vi "iRFMeasureAuto.vi"() -> ()   [LabVIEW 2019]
uses:
  SubVI/LabJack/LJ Pin Setting.ctl
  SubVI/LabJack/LJ PWM Setting.ctl
  <instrlib>/niScope/Controls/niScope vertical coupling.ctl
  <instrlib>/niScope/Controls/niScope trigger source.ctl
  <vilib>/Analysis/baseanly.llb/Mean (DBL).vi
  <instrlib>/niScope/Configure/Trigger/niScope Configure Trigger Edge.vi
  <instrlib>/niScope/Acquire/Fetch/niScope Fetch.vi
  <instrlib>/niScope/Acquire/Fetch/niScope Multi Fetch.vi
  <vilib>/Analysis/NI_AALBase.lvlib
panel:
  in  "Prefix":string
  out "Current State":string
  out "Exit Try":bool
  in  "Suffix":string
  out "355nm Laser":bool
  out "laser EM lamp V":dbl format="%0.6f"
  in  "Aquire":bool
  in  "Current V":dbl min=0.0 max=4.7 step=0.1
  out "error out":errorcluster
  in  "Live":bool=TRUE
  out "Waveform Graph":dbl[](graph)
  in  "Channel":enum16{"Ch1", "Ch2", "Ch3"}(ring)
  in  "OK":bool
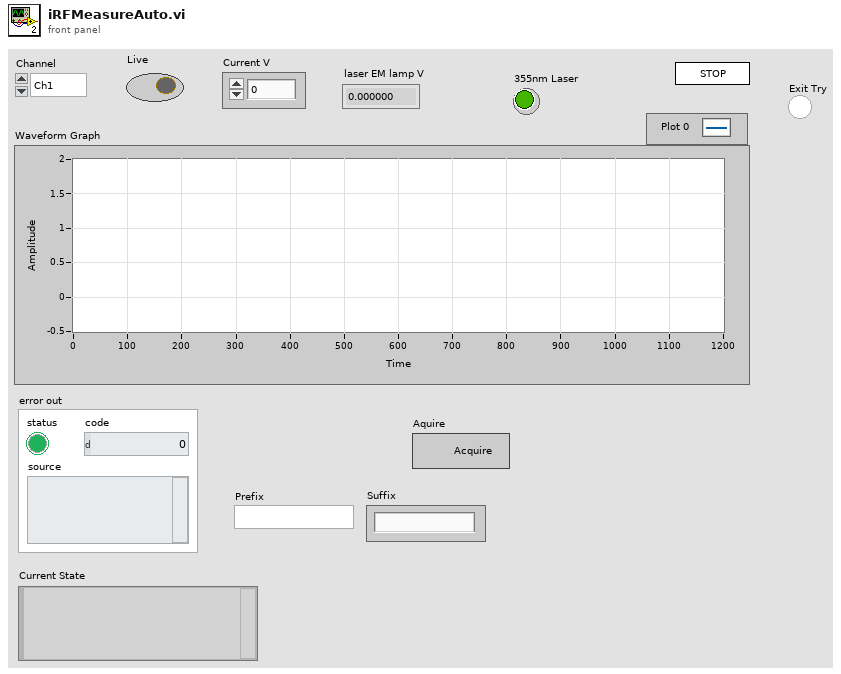
[diagram p1: front panel]
types:
  T1 = enum32{"Invalid", "Standard", "Closed", "Hidden", "Minimized", "Maximized"}
  T2 = enum32{"invalid app kind", "Development System", "Run Time System", "Student Edition", "Embedded LabVIEW", "Evaluation", "Custom"}
  T3 = typedef "niScope trigger source.ctl" = string
  T4 = enum16{"open", "open or create", "create or replace", "create", "open (read-only)"}
  T5 = typedef "LJ Pin Setting.ctl" = cluster{"Ch1 Bias":string, "Ch2 Bias":string, "Ch3 Bias":string, "355 PWM":string, "AimingBeam PWM":string, "Laser Ready":string, "Interlock":string, "Laser Start/Stop":string, "Red LED":string, "Green LED":string, "Foot Pedal":string}
  T6 = typedef "LJ PWM Setting.ctl" = cluster{"DIO_EF_CLOCK1_DIVISOR":i16, "DIO_EF_CLOCK1_ROLL_VALUE":i32, "DIO#_EF_INDEX":i16, "DIO#_EF_OPTIONS":i16, "DIO#_EF_CONFIG_A":i32}
  T7 = cluster{"Core":cluster{"Current VI Reference":refnum<vi>, "Close Panel on Exit?":bool}, "355 Status":bool, "Your string data":string, "Channel":enum16{"Ch1", "Ch2", "Ch3"}, "Digitizer":refnum<k15>, "Dig channels":string, "num points":i32, "LJ Handle":i32, "LJ pin":string, "V":dbl, "wfm":dbl[][], "LJ Pins":T5, "PWM Setting":T6, "Exit Try":bool}
  T8 = cluster{"Current VI Reference":refnum<vi>, "Close Panel on Exit?":bool}
  T9 = typedef "niScope vertical coupling.ctl" = i32
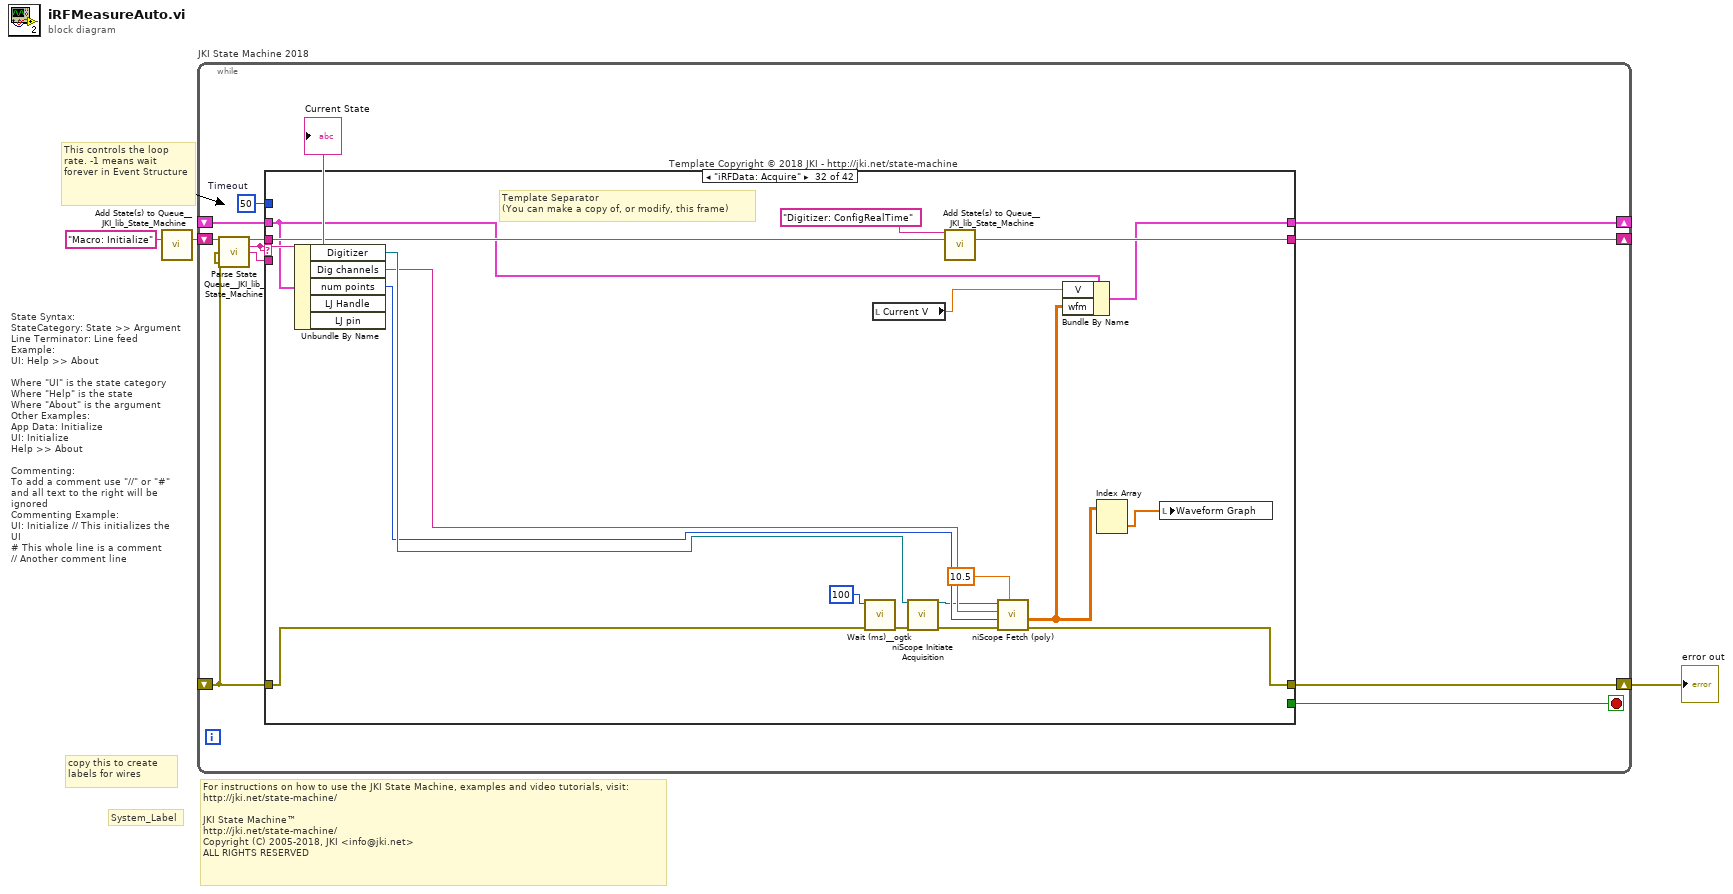
[diagram p0: block diagram]
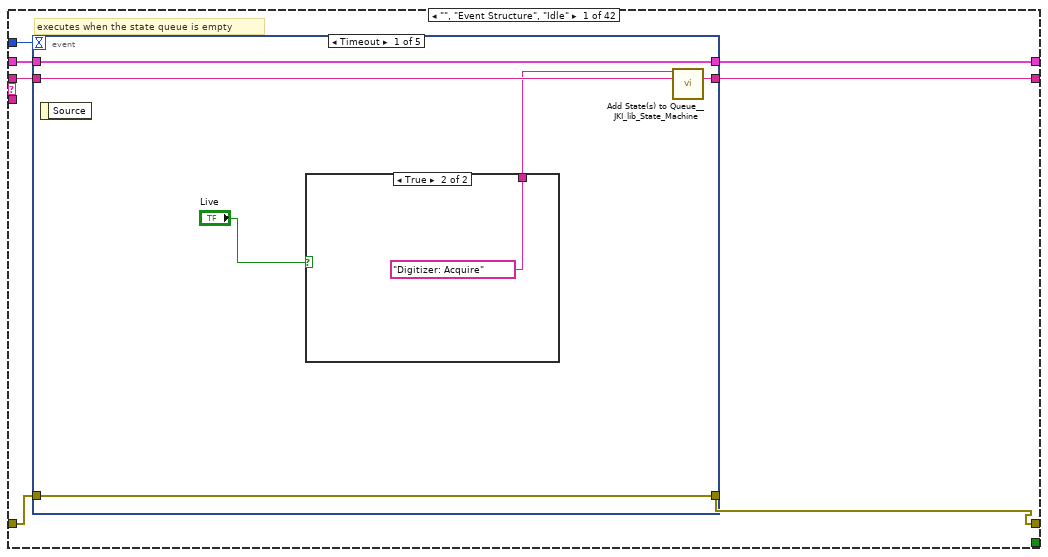
[diagram p2: hidden frame]
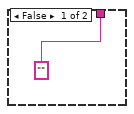
[diagram p3: hidden frame]
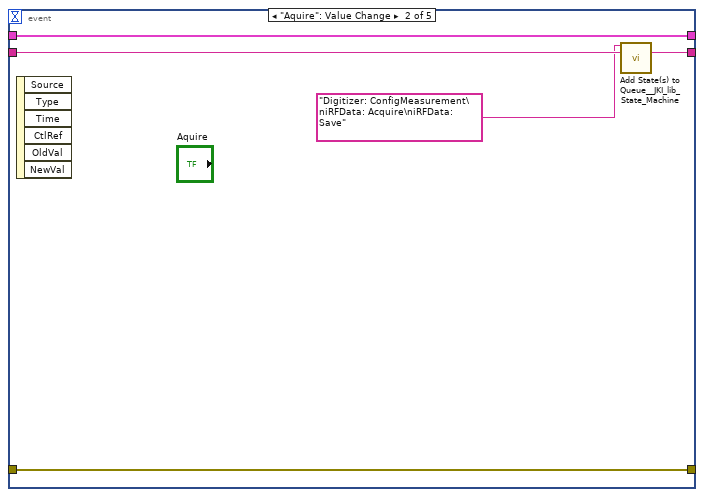
[diagram p4: hidden frame]
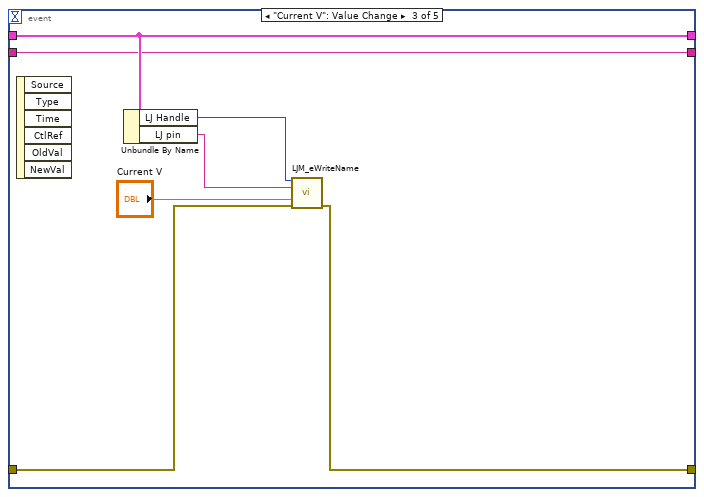
[diagram p5: hidden frame]
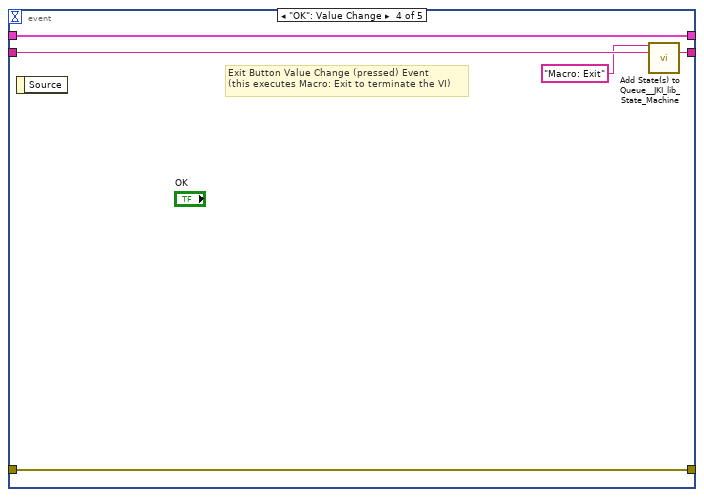
[diagram p6: hidden frame]
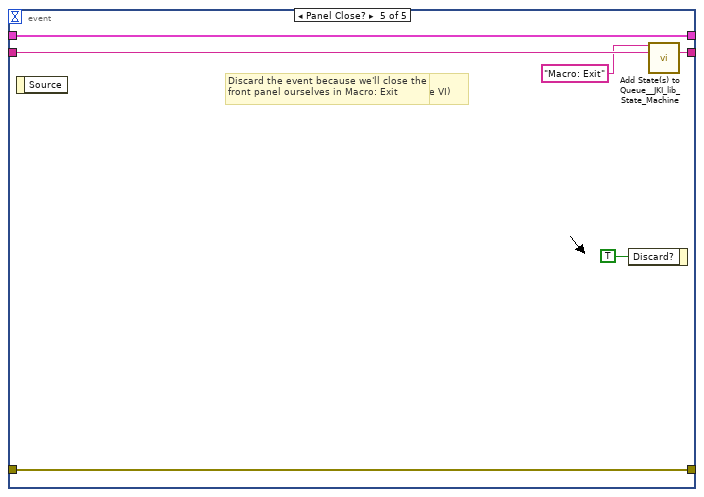
[diagram p7: hidden frame]
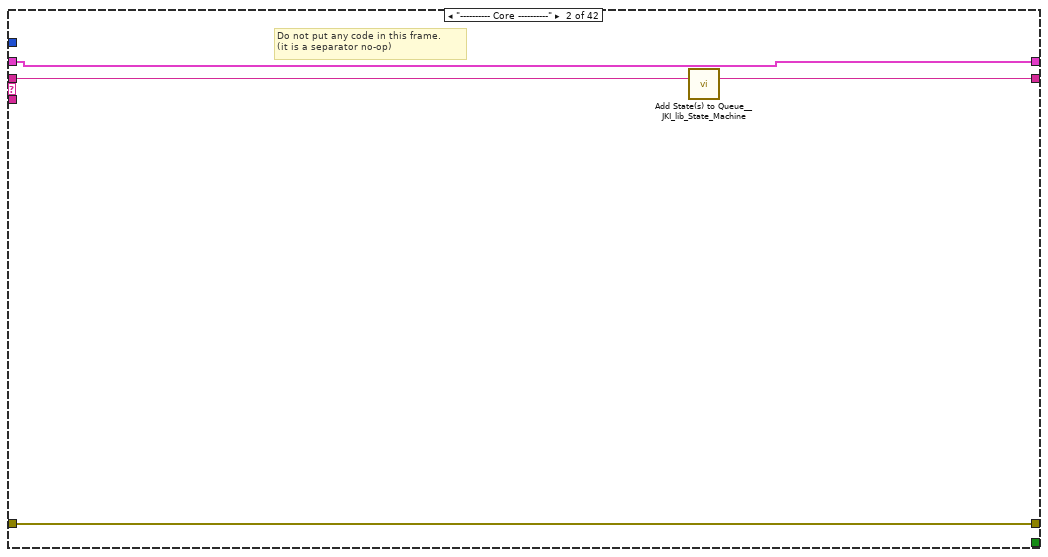
[diagram p8: hidden frame]
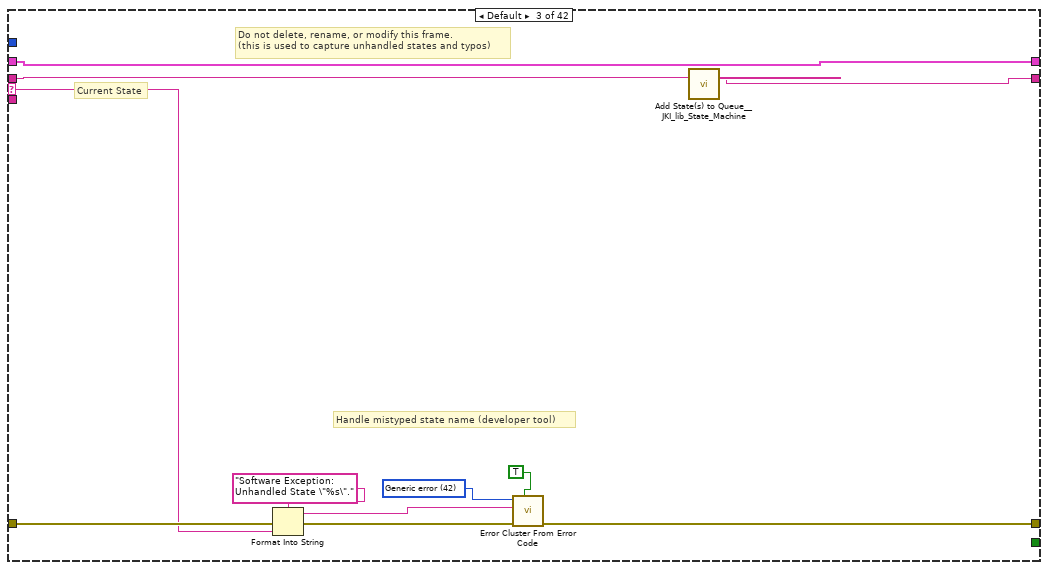
[diagram p9: hidden frame]
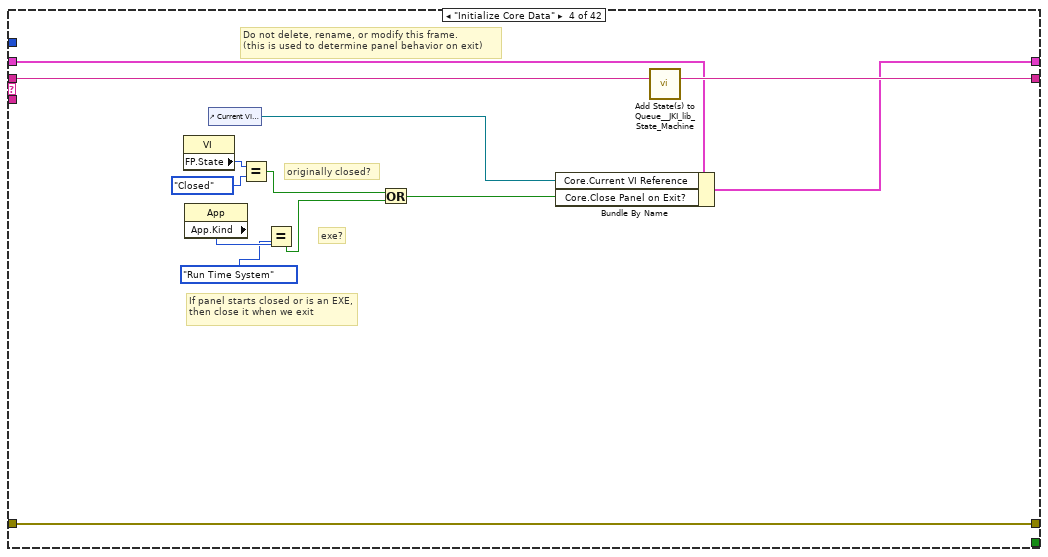
[diagram p10: hidden frame]
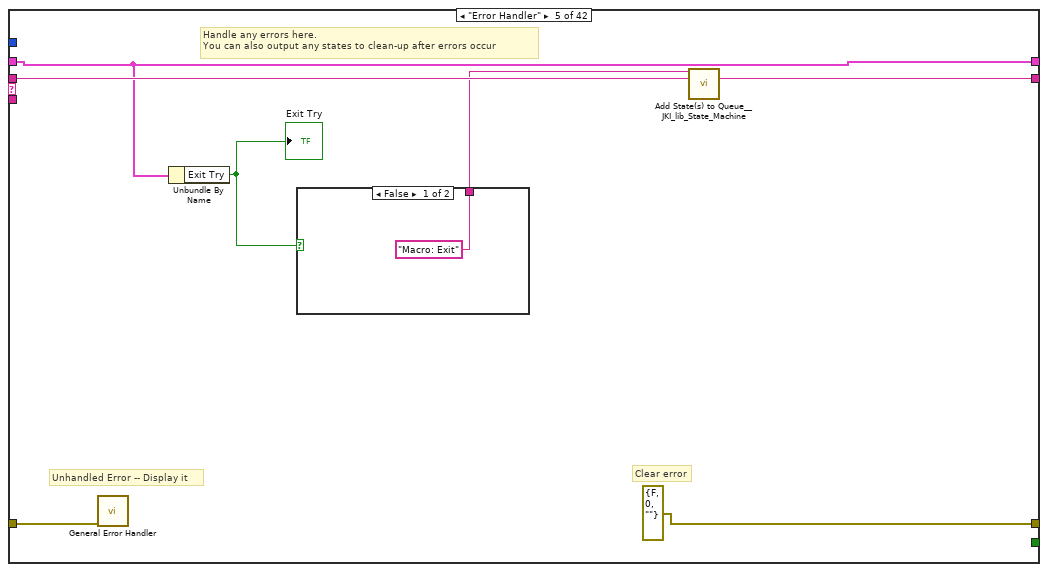
[diagram p11: hidden frame]
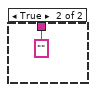
[diagram p12: hidden frame]
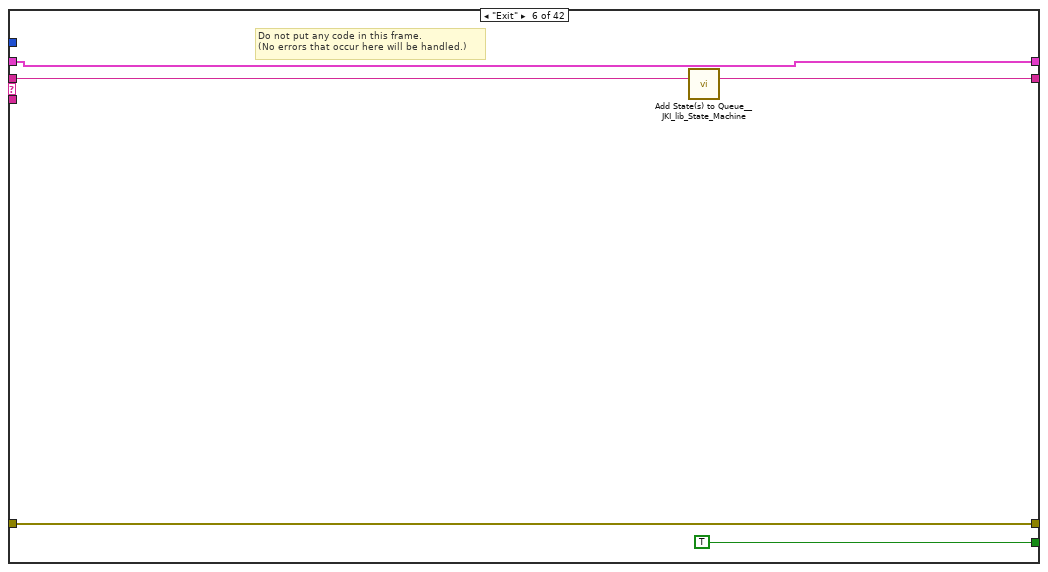
[diagram p13: hidden frame]
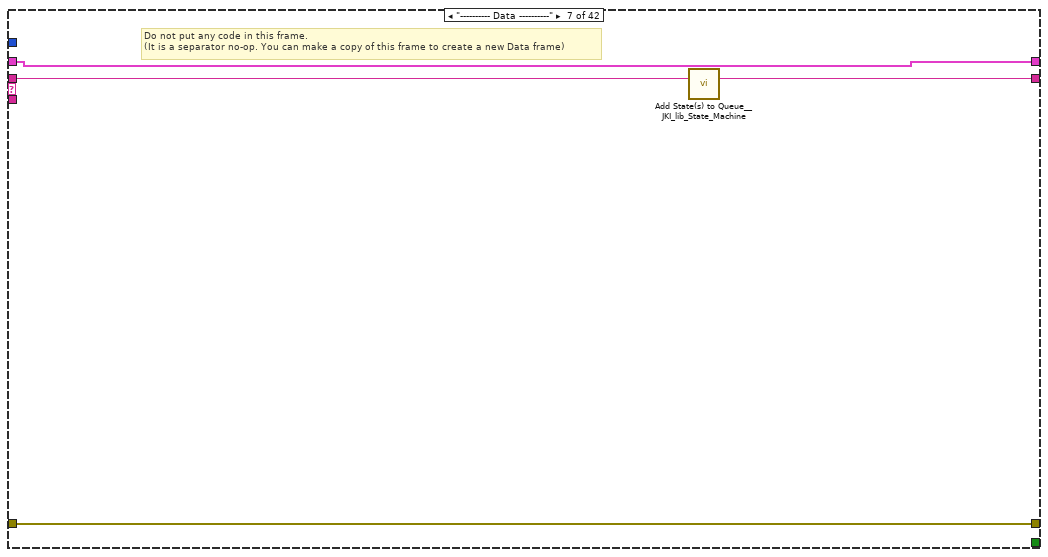
[diagram p14: hidden frame]
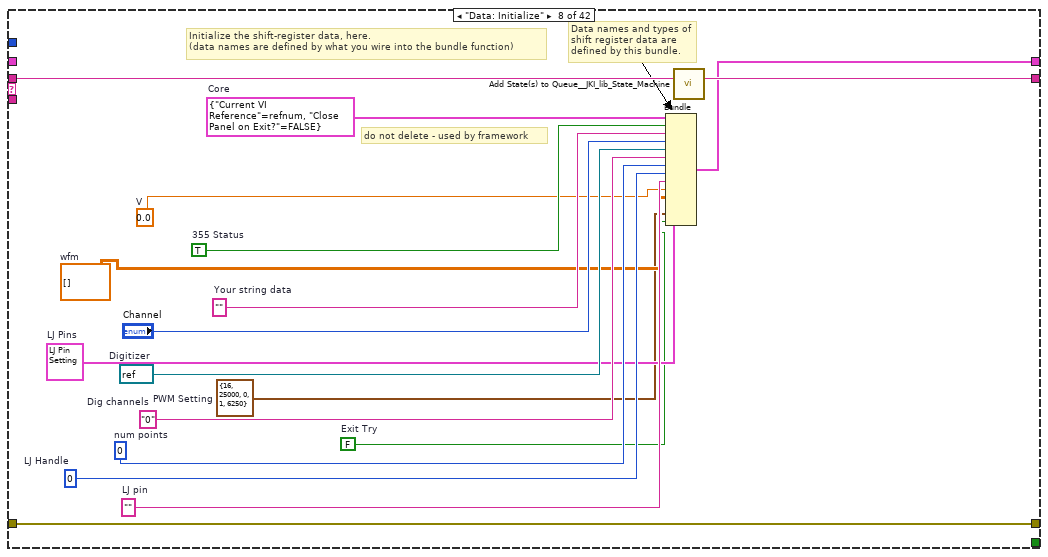
[diagram p15: hidden frame]
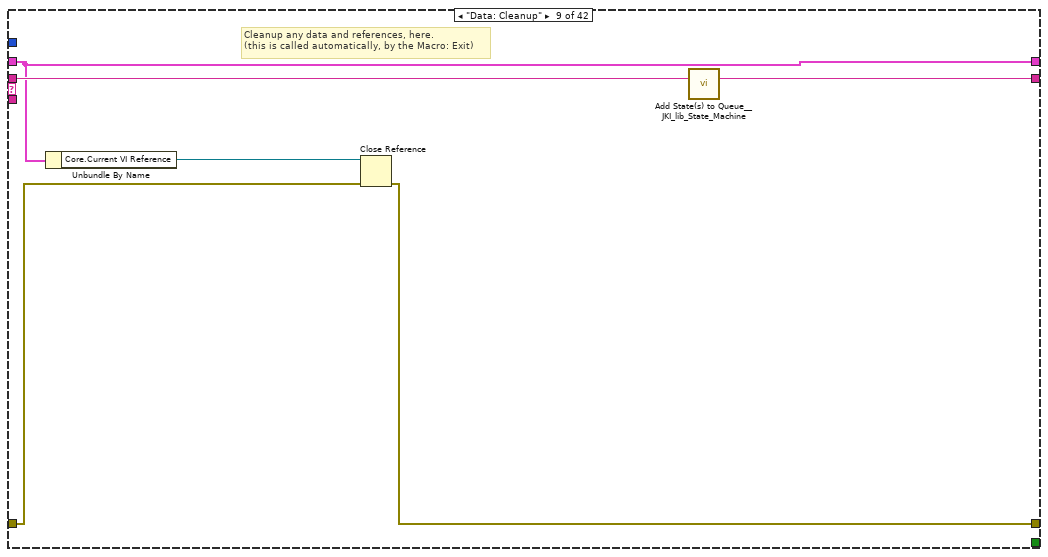
[diagram p16: hidden frame]
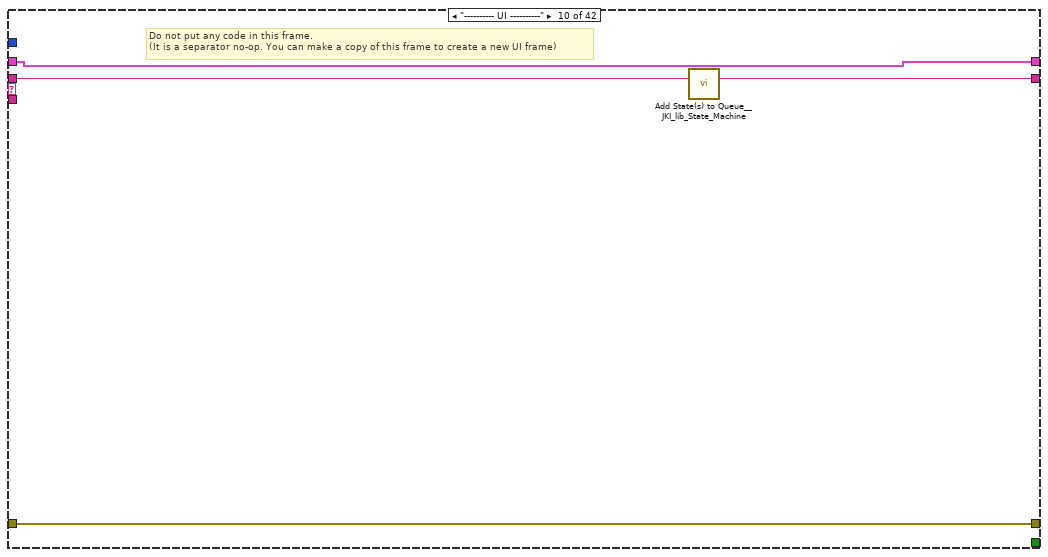
[diagram p17: hidden frame]
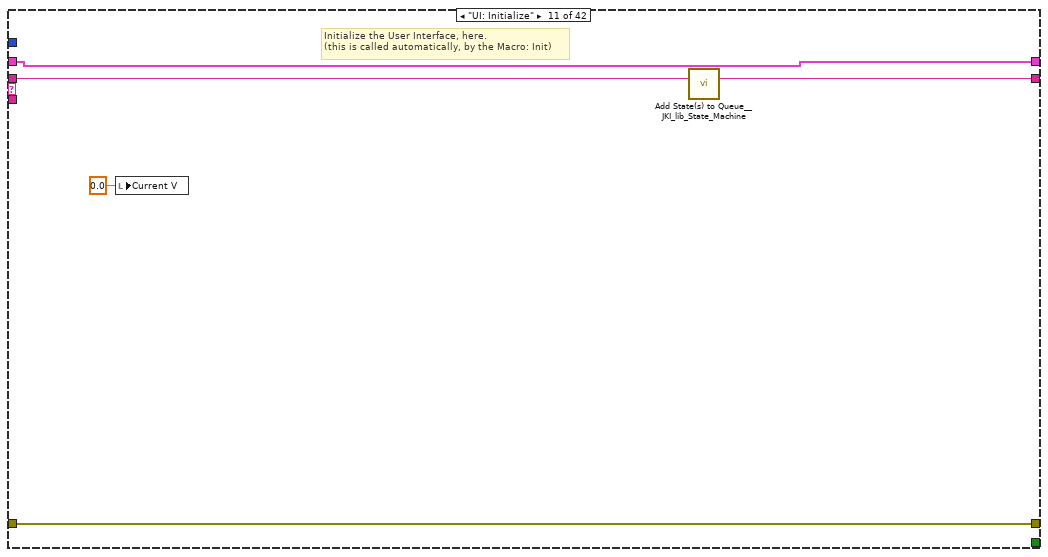
[diagram p18: hidden frame]
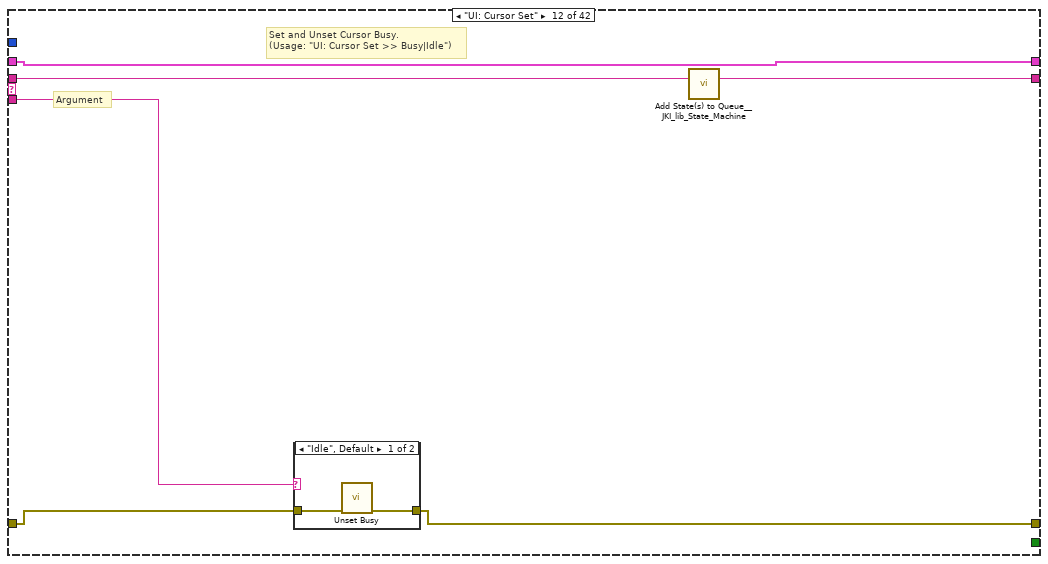
[diagram p19: hidden frame]
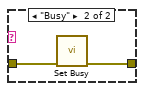
[diagram p20: hidden frame]
diagram:
  # "For instructions on how to use the JKI State Machine, examples and video tutorials, visit:\nhttp://jki.net/state-machine/\n\nJKI State Machine™\nhttp://jki.net/state-machine/\nCopyright (C) 2005-2018, JKI <info@jki.net>\nALL RIGHTS RESERVED"
  # "State Syntax:\nStateCategory: State >> Argument\nLine Terminator: Line feed\nExample:\nUI: Help >> About\n\nWhere \"UI\" is the state category\nWhere \"Help\" is the state\nWhere \"About\" is the argument\nOther Examples:\nApp Data: Initialize\nUI: Initialize\nHelp >> About\n\nCommenting:\nTo add a comment use \"//\" or \"#\" and all text to the right will be ignored\nCommenting Example:\nUI: Initialize // This initializes the UI\n# This whole line is a comment\n// Another comment line"
  # "copy this to create labels for wires"
  # "This controls the loop rate. -1 means wait forever in Event Structure"
  # "System_Label"
  n1 = call <vilib>:"Add State(s) to Queue__JKI_lib_State_Machine.vi"("State(s) in (\"\")"="Macro: Initialize") -> ("States Out"=w3:string)  [unwired: 14 in]
  n2 = while "JKI State Machine 2018" {
    shift-right: [w7] -> _
    shift-left: _ -> [w6]
    shift-right: [w10] -> w1
    shift-left: _ -> [w4]
    shift-right: [w9] -> _
    shift-left: w3 -> [w11]
    stop <- w8 stop-if-true
    w5 = 50  # Timeout
    # "Template Copyright © 2018 JKI - http://jki.net/state-machine"
    n3 = call <vilib>:"Parse State Queue__JKI_lib_State_Machine.vi"("State Queue"=w11, "Error In (no error)"=w4) -> ("Remaining States"=w13:string, "Current State"=w14:string, "Arguments"=w12:string)  [unwired: 11 in]
    "Current State" <- w14
    n4 = case shown="\"iRFData: Acquire\"" w14 {
      selector: w14 -> [_ _ w57 _ _ _ _ _ _ _ _ _ _ _ _ _ _ _ _ _ _ _ _ _ _ _ _ _ _ _ _ _ _ _ _ _ _ _ _ _ _ _]
      tunnel: w13 -> [w21 w56 w61 w80 w87 w94 w98 w116 w122 w126 w131 w137 w148 w217 w222 w234 w238 w247 w265 w300 w341 w358 w375 w379 w388 w417 w424 w433 w441 w447 w451 w469 w502 w511 w523 w561 w571 w580 w600 w616 w620 w624]
      tunnel: w12 -> [_ _ _ _ _ _ _ _ _ _ _ w132 w142 _ _ _ _ _ _ _ _ _ _ _ _ _ _ _ _ _ _ _ _ _ _ _ _ _ _ _ _ _]
      tunnel: w6 -> [w19 w53 w59 w73 w83 w92 w95 _ w117 w123 w129 w135 w144 w214 w219 w224 w235 w239 w261 w288 w329 w356 w373 w376 w381 w389 w419 w426 w439 w445 w448 w461 w479 w508 w514 w555 w565 w576 w596 w613 w617 w621]
      tunnel: [w18 w54 w63 w77 errorcluster {"status"=FALSE, "code"=0, "source"=""} ("error out") w91 w96 w113 w118 w124 w128 w133 w145 w215 w220 w232 w236 w245 w263 w281 w322 w353 w369 w377 w386 w391 w422 w431 w435 w443 w449 w463 w485 w509 w516 w553 w563 w573 w594 w614 w618 w622] -> w10
      tunnel: w4 -> [w17 w54 w62 w77 w84 w91 w96 w113 w119 w124 w128 w134 w146 w215 w220 w232 w236 w245 w262 w275 w316 w350 w368 w377 w386 w392 w421 w431 w434 w442 w449 w464 w484 w509 w516 w552 w562 w574 w593 w614 w618 w622]
      tunnel: [w20 w55 w60 w79 w86 w93 w97 w115 w121 w125 w130 w136 w147 w216 w221 w233 w237 w246 w264 w299 w340 w357 w374 w378 w387 w416 w423 w432 w440 w446 w450 w468 w501 w510 w522 w560 w570 w579 w599 w615 w619 w623] -> w9
      tunnel: [_ _ _ _ _ TRUE _ _ _ _ _ _ _ _ _ _ _ _ _ _ _ _ _ _ _ _ _ _ _ _ _ _ _ _ _ _ _ _ _ _ _ _] -> w8
      tunnel: [w16 w53 w59 w78 w83 w92 w95 w114 w117 w123 w129 w135 w144 w214 w219 w225 w235 w242 w261 w289 w330 w356 w373 w376 w382 w389 w420 w427 w439 w445 w448 w462 w479 w508 w515 w555 w565 w576 w596 w613 w617 w621] -> w7
      tunnel: w5 -> [w15 _ _ _ _ _ _ _ _ _ _ _ _ _ _ _ _ _ _ _ _ _ _ _ _ _ _ _ _ _ _ _ _ _ _ _ _ _ _ _ _ _]
      frame "", "Event Structure", "Idle" {
        # "executes when the state queue is empty"
        n5 = event shown="[0] Timeout" {
          selector: _ -> [_ _ _ _ _]
          dyn-events: _ -> [_ _ _ _ _]
          timeout: w15 -> [_ _ _ _ _]
          tunnel: w21 -> [w27 w32 w35 w46 w52]
          tunnel: [w26 w33 w35 w45 w51] -> w20
          tunnel: w19 -> [w24 w34 w36 w43 w49]
          tunnel: [w25 w30 w37 w44 w50] -> w18
          tunnel: w17 -> [w25 w30 w38 w44 w50]
          tunnel: [w24 w34 w36 w43 w49] -> w16
          event Timeout {
            n6 = event-data() -> ()  [unwired: 1 in, 1 out]
            n7 = case shown="True" "Live" {
              tunnel: ["" ("State(s) in Front (\"\")") "Digitizer: Acquire" ("State(s) in Front (\"\")")] -> w22
              frame False {
              }
              frame True {
              }
            }
            n8 = call <vilib>:"Add State(s) to Queue__JKI_lib_State_Machine.vi"("State(s) in Front (\"\")"=w22, "State(s) in (\"\")"=w27) -> ("States Out"=w26:string)  [unwired: 13 in]
          }
          event "Aquire": Value Change {
            n9 = event-data() -> ()  [unwired: 1 in, 6 out]
            n10 = call <vilib>:"Add State(s) to Queue__JKI_lib_State_Machine.vi"("State(s) in Front (\"\")"="Digitizer: ConfigMeasurement\niRFData: Acquire\niRFData: Save" ("States Out"), "State(s) in (\"\")"=w32) -> ("States Out"=w33:string)  [unwired: 13 in]
          }
          event "Current V": Value Change {
            n11 = event-data() -> ()  [unwired: 1 in, 6 out]
            n12 = Unbundle By Name(w36) -> ("LJ Handle"=w41:i32, "LJ pin"=w40:string)
            n13 = call <vilib>:"LJM_eWriteName.vi"("Handle In"=w41, "Name"=w40, "Value"="Current V", "error in"=w38) -> ("error out"=w37:errorcluster)  [unwired: 10 in, 1 out]
          }
          event "OK": Value Change {
            # "Exit Button Value Change (pressed) Event\n(this executes Macro: Exit to terminate the VI)"
            n14 = event-data() -> ()  [unwired: 1 in, 1 out]
            n15 = call <vilib>:"Add State(s) to Queue__JKI_lib_State_Machine.vi"("State(s) in Front (\"\")"="Macro: Exit", "State(s) in (\"\")"=w46) -> ("States Out"=w45:string)  [unwired: 13 in]
          }
          event Panel Close? {
            # "Discard the event because we'll close the front panel ourselves in Macro: Exit"
            # "Close Panel button (pressed) Event\n(this executes Macro: Exit to terminate the VI)"
            n16 = event-data() -> ()  [unwired: 1 in, 1 out]
            n17 = event-data("Discard?"=TRUE) -> ()  [unwired: 1 in, 1 out]
            n18 = call <vilib>:"Add State(s) to Queue__JKI_lib_State_Machine.vi"("State(s) in Front (\"\")"="Macro: Exit", "State(s) in (\"\")"=w52) -> ("States Out"=w51:string)  [unwired: 13 in]
          }
        }
      }
      frame "---------- Core ----------" {
        # "Do not put any code in this frame.\n(it is a separator no-op)"
        n19 = call <vilib>:"Add State(s) to Queue__JKI_lib_State_Machine.vi"("State(s) in (\"\")"=w56) -> ("States Out"=w55:string)  [unwired: 14 in]
      }
      frame Default {
        w66 = 42 items=["No error", "Argument error", "Memory is full", "Out of zone", "End of file", "File already open", "Generic file I/O error", "File not found", "File permission error", "Disk is full", "Duplicate path", "Too many files open", "System feature not enabled", "Resource file not found", "Cannot add resource", "Resource not found", "Image not found", "Image memory error", "Pen does not exist", "Config type invalid", "Config token not found", "Config parse error", "Config memory error", "Bad external code format", "Bad external code offset", "External code not present", "Null window", "Destroy window error", "Null menu", "Print aborted", "Bad print record", "Print driver error", "Windows error during printing", "Memory error during printing", "Print dialog error", "Generic print error", "Invalid device refnum", "Device not found", "Device parameter error", "Device unit error", "Cannot open device", "Device call aborted", "Generic error", "Cancelled by user", "Object ID too low", "Object ID too high", "Object not in heap", "Unknown heap", "Unknown object (invalid DefProc)", "Unknown object (DefProc not in table)", "Message out of range", "Invalid (null) method", "Unknown message", "Manager call not supported", "Bad address", "Network operation in progress", "Network operation timed out", "Connection is busy", "Network attribute not supported", "Network error", "Address in use", "System out of memory", "Connection aborted", "Connection refused", "Not connected", "Already connected", "Connection closed", "Initialization error (interapplication manager)", "Bad occurrence", "Wait on unbound occurrence handler", "Occurrence queue overflow", "Datalog type conflict", "Unused", "Unrecognized type (interapplication manager)", "Memory corrupt", "Failed to make temporary DLL", "Old CIN version", "Drag socket not found", "Failed to load drop-object", "Failed to register OLE object", "Failed to release OLE object", "Format specifier type mismatch", "Unknown format specifier", "Too few format specifiers", "Too many format specifiers", "Scan failed", "Newer CIN version", "Error converting to variant", "Runtime menu error", "Password tampered", "Variant attribute not found", "Incompatible variant data type", "Event data is not available", "Event Store is not present", "Occurrence is not found", "Event Queue is not created", "Event info is not available", "Refnum passed is NULL", "Error retrieving Class GUID", "Error retrieving CoClass GUID", "Error retrieving TypeLib GUID.", "Bad built application magic bytes.", "Specific driver is different from the specific driver associated with the Logical Name.", "There is no session opened to the class driver.", "Max Error", "MAX - Error with config objects", "MAX - Error loading configuration", "MAX - Group not supported"]
        # "Current State"
        # "Do not delete, rename, or modify this frame.\n(this is used to capture unhandled states and typos)"
        # "Handle mistyped state name (developer tool)"
        n20 = Format Into String(format string="Software Exception: Unhandled State \"%s\"." ("message"), error in=w62, w57) -> (resulting string=w65:string, error out=w64:errorcluster)  [unwired: 1 in]
        n21 = call <vilib>:"Error Cluster From Error Code.vi"("show call chain? (False)"=TRUE, "error in (no error)"=w64, "error message (\"\")"=w65, "error code (0)"=w66) -> ("error out"=w63:errorcluster)  [unwired: 5 in]
        n22 = call <vilib>:"Add State(s) to Queue__JKI_lib_State_Machine.vi"("State(s) in (\"\")"=w61) -> ("States Out"=w60:string)  [unwired: 14 in]
      }
      frame "Initialize Core Data" {
        # "Do not delete, rename, or modify this frame.\n(this is used to determine panel behavior on exit)"
        # "originally closed?"
        # "exe?"
        # "If panel starts closed or is an EXE, then close it when we exit"
        n23 = property class="VI"() -> ("FP.State"=w70:T1)  [unwired: 2 in, 2 out]
        n24 = property class="App"() -> ("App.Kind"=w76:T2)  [unwired: 2 in, 2 out]
        n25 = control-ref of="Current VI Reference"() -> (w71:refnum<vi>)
        n26 = Equal?(x=w70, y=T1."Closed" ("Front Panel Window:State")) -> (x = y?=w68:bool)
        n27 = Equal?(x=w76, y=T2."Run Time System" ("Application:Kind")) -> (x = y?=w74:bool)
        n28 = Or(x=w68, y=w74) -> (x .or. y?=w72:bool)
        n29 = Bundle By Name(cluster=w73, "Core.Current VI Reference"=w71, "Core.Close Panel on Exit?"=w72) -> (w78:T7)
        n30 = call <vilib>:"Add State(s) to Queue__JKI_lib_State_Machine.vi"("State(s) in (\"\")"=w80) -> ("States Out"=w79:string)  [unwired: 14 in]
      }
      frame "Error Handler" {
        # "Unhandled Error -- Display it"
        # "Handle any errors here.\nYou can also output any states to clean-up after errors occur"
        # "Clear error"
        n31 = call <vilib>:"General Error Handler.vi"("error in (no error)"=w84) -> ()  [unwired: 10 in, 5 out]
        n32 = Unbundle By Name(w83) -> ("Exit Try"=w82:bool)
        "Exit Try" <- w82
        n33 = case shown="False" w82 {
          tunnel: ["Macro: Exit" ""] -> w81
          frame False {
          }
          frame True {
          }
        }
        n34 = call <vilib>:"Add State(s) to Queue__JKI_lib_State_Machine.vi"("State(s) in Front (\"\")"=w81, "State(s) in (\"\")"=w87) -> ("States Out"=w86:string)  [unwired: 13 in]
      }
      frame "Exit" {
        # "Do not put any code in this frame.\n(No errors that occur here will be handled.)"
        n35 = call <vilib>:"Add State(s) to Queue__JKI_lib_State_Machine.vi"("State(s) in (\"\")"=w94) -> ("States Out"=w93:string)  [unwired: 14 in]
      }
      frame "---------- Data ----------" {
        # "Do not put any code in this frame.\n(It is a separator no-op. You can make a copy of this frame to create a new Data frame)"
        n36 = call <vilib>:"Add State(s) to Queue__JKI_lib_State_Machine.vi"("State(s) in (\"\")"=w98) -> ("States Out"=w97:string)  [unwired: 14 in]
      }
      frame "Data: Initialize" {
        w99 = FALSE  # Exit Try
        w100 = T6 {"DIO_EF_CLOCK1_DIVISOR"=16, "DIO_EF_CLOCK1_ROLL_VALUE"=25000, "DIO#_EF_INDEX"=0, "DIO#_EF_OPTIONS"=1, "DIO#_EF_CONFIG_A"=6250}  # PWM Setting
        w101 = T5 {"Ch1 Bias"="TDAC13", "Ch2 Bias"="TDAC12", "Ch3 Bias"="DAC0", "355 PWM"="DIO2", "AimingBeam PWM"="DIO3", "Laser Ready"="AIN0", "Interlock"="NOT USED", "Laser Start/Stop"="DIO8", "Red LED"="TDAC10", "Green LED"="TDAC11", "Foot Pedal"="DIO14"}  # LJ Pins
        w102 = dbl[][] []  # wfm
        w103 = 0.0  # V
        w104 = ""  # LJ pin
        w105 = 0  # LJ Handle
        w106 = 0  # num points
        w107 = "0"  # Dig channels
        w108 = refnum<k15> refnum  # Digitizer
        w110 = T8 {"Current VI Reference"=refnum, "Close Panel on Exit?"=FALSE}  # Core
        w112 = TRUE  # 355 Status
        w111 = ""  # Your string data
        # "do not delete - used by framework"
        # "Data names and types of shift register data are defined by this bundle."
        # "Initialize the shift-register data, here.\n(data names are defined by what you wire into the bundle function)"
        n37 = Bundle("Core"=w110, "355 Status"=w112, "Your string data"=w111, "Channel"="Channel", "Digitizer"=w108, "Dig channels"=w107, "num points"=w106, "LJ Handle"=w105, "LJ pin"=w104, "V"=w103, "wfm"=w102, "LJ Pins"=w101, "PWM Setting"=w100, "Exit Try"=w99) -> (w114:T7)  [unwired: 1 in]
        n38 = call <vilib>:"Add State(s) to Queue__JKI_lib_State_Machine.vi"("State(s) in (\"\")"=w116) -> ("States Out"=w115:string)  [unwired: 14 in]
      }
      frame "Data: Cleanup" {
        # "Cleanup any data and references, here.\n(this is called automatically, by the Macro: Exit)"
        n39 = Unbundle By Name(w117) -> ("Core.Current VI Reference"=w120:refnum<vi>)
        n40 = Close Reference(reference=w120, error in (no error)=w119) -> (error out=w118:errorcluster)
        n41 = call <vilib>:"Add State(s) to Queue__JKI_lib_State_Machine.vi"("State(s) in (\"\")"=w122) -> ("States Out"=w121:string)  [unwired: 14 in]
      }
      frame "---------- UI ----------" {
        # "Do not put any code in this frame.\n(It is a separator no-op. You can make a copy of this frame to create a new UI frame)"
        n42 = call <vilib>:"Add State(s) to Queue__JKI_lib_State_Machine.vi"("State(s) in (\"\")"=w126) -> ("States Out"=w125:string)  [unwired: 14 in]
      }
      frame "UI: Initialize" {
        # "Initialize the User Interface, here.\n(this is called automatically, by the Macro: Init)"
        n43 = local write "Current V"(0.0 ("Current V")) -> ()
        n44 = call <vilib>:"Add State(s) to Queue__JKI_lib_State_Machine.vi"("State(s) in (\"\")"=w131) -> ("States Out"=w130:string)  [unwired: 14 in]
      }
      frame "UI: Cursor Set" {
        # "Argument"
        # "Set and Unset Cursor Busy.\n(Usage: \"UI: Cursor Set >> Busy|Idle\")"
        n45 = case shown="\"Idle\", Default" w132 {
          tunnel: w134 -> [w139 w141]
          tunnel: [w138 w140] -> w133
          frame "Idle", Default {
            n46 = call <vilib>:"Unset Busy.vi"("error in (no error)"=w139) -> ("error out"=w138:errorcluster)  [unwired: 10 in]
          }
          frame "Busy" {
            n47 = call <vilib>:"Set Busy.vi"("error in (no error)"=w141) -> ("error out"=w140:errorcluster)  [unwired: 9 in, 1 out]
          }
        }
        n48 = call <vilib>:"Add State(s) to Queue__JKI_lib_State_Machine.vi"("State(s) in (\"\")"=w137) -> ("States Out"=w136:string)  [unwired: 14 in]
      }
      frame "UI: Front Panel State" {
        # "Argument"
        # "Set Front Panel Open or Closed\n(Usage: \"UI: Front Panel State >> Open|Close\")"
        n49 = Unbundle By Name(w144) -> ("Core.Current VI Reference"=w143:refnum<vi>)
        n50 = case shown="\"Minimize\", \"Minimized\"" w142 {
          tunnel: w146 -> [w154 w169 w180 w193 w206]
          tunnel: [w156 w170 w182 w195 w208] -> w145
          tunnel: w143 -> [w155 w167 w181 w194 w207]
          frame "Open", "Standard", Default {
            w149 = T1."Standard" ("State")
            n51 = property class="VI"(reference=w155, error in=w154) -> (reference out=w152:refnum<vi>, error out=w153:errorcluster, "FP.State"=w151:T1)
            n52 = Not Equal?(x=w151, y=w149) -> (x != y?=w150:bool)
            n53 = case shown="True" w150 {
              tunnel: [w160 w162] -> w156
              tunnel: w153 -> [w159 w162]
              tunnel: w152 -> [w158 _]
              tunnel: w149 -> [w157 _]
              frame True {
                n54 = invoke class="VI" method="FP.Open"(reference=w158, error in=w159, "Activate"=TRUE, "State"=w157) -> (error out=w160:errorcluster)  [unwired: 1 in, 4 out]
              }
              frame False {
              }
            }
          }
          frame "Close", "Closed" {
            n55 = property class="VI"(reference=w167, error in=w169) -> (reference out=w166:refnum<vi>, error out=w168:errorcluster, "FP.State"=w164:T1)
            n56 = Not Equal?(x=w164, y=T1."Closed" ("Front Panel Window:State")) -> (x != y?=w163:bool)
            n57 = case shown="True" w163 {
              tunnel: [w171 w174] -> w170
              tunnel: w168 -> [w171 w173]
              tunnel: w166 -> [_ w172]
              frame False {
              }
              frame True {
                n58 = invoke class="VI" method="FP.Close"(reference=w172, error in=w173) -> (error out=w174:errorcluster)  [unwired: 1 in, 2 out]
              }
            }
          }
          frame "Hidden", "Hide" {
            w175 = T1."Hidden" ("State")
            n59 = property class="VI"(reference=w181, error in=w180) -> (reference out=w178:refnum<vi>, error out=w179:errorcluster, "FP.State"=w177:T1)
            n60 = Not Equal?(x=w177, y=w175) -> (x != y?=w176:bool)
            n61 = case shown="True" w176 {
              tunnel: [w186 w187] -> w182
              tunnel: w179 -> [w185 w187]
              tunnel: w178 -> [w184 _]
              tunnel: w175 -> [w183 _]
              frame True {
                n62 = invoke class="VI" method="FP.Open"(reference=w184, error in=w185, "State"=w183) -> (error out=w186:errorcluster)  [unwired: 2 in, 4 out]
              }
              frame False {
              }
            }
          }
          frame "Minimize", "Minimized" {
            w188 = T1."Minimized" ("State")
            n63 = property class="VI"(reference=w194, error in=w193) -> (reference out=w191:refnum<vi>, error out=w192:errorcluster, "FP.State"=w190:T1)
            n64 = Not Equal?(x=w190, y=w188) -> (x != y?=w189:bool)
            n65 = case shown="True" w189 {
              tunnel: [w199 w200] -> w195
              tunnel: w192 -> [w198 w200]
              tunnel: w191 -> [w197 _]
              tunnel: w188 -> [w196 _]
              frame True {
                n66 = invoke class="VI" method="FP.Open"(reference=w197, error in=w198, "State"=w196) -> (error out=w199:errorcluster)  [unwired: 2 in, 4 out]
              }
              frame False {
              }
            }
          }
          frame "Maximize", "Maximized" {
            w201 = T1."Maximized" ("State")
            n67 = property class="VI"(reference=w207, error in=w206) -> (reference out=w204:refnum<vi>, error out=w205:errorcluster, "FP.State"=w203:T1)
            n68 = Not Equal?(x=w203, y=w201) -> (x != y?=w202:bool)
            n69 = case shown="True" w202 {
              tunnel: [w212 w213] -> w208
              tunnel: w205 -> [w211 w213]
              tunnel: w204 -> [w210 _]
              tunnel: w201 -> [w209 _]
              frame True {
                n70 = invoke class="VI" method="FP.Open"(reference=w210, error in=w211, "State"=w209) -> (error out=w212:errorcluster)  [unwired: 2 in, 4 out]
              }
              frame False {
              }
            }
          }
        }
        n71 = call <vilib>:"Add State(s) to Queue__JKI_lib_State_Machine.vi"("State(s) in (\"\")"=w148) -> ("States Out"=w147:string)  [unwired: 14 in]
      }
      frame "---------- Macro ----------" {
        # "Do not put any code in this frame.\n(It is a separator no-op. You can make a copy of this frame to create a new Macro frame)"
        n72 = call <vilib>:"Add State(s) to Queue__JKI_lib_State_Machine.vi"("State(s) in (\"\")"=w217) -> ("States Out"=w216:string)  [unwired: 14 in]
      }
      frame "Macro: Initialize" {
        # "Initialization Macro\n(This is called once, when the VI starts)"
        n73 = call <vilib>:"Add State(s) to Queue__JKI_lib_State_Machine.vi"("State(s) in Front (\"\")"="Data: Initialize\nInitialize Core Data\nUI: Initialize\nUI: Front Panel State >> Open\nDigitizer: Select\nDigitizer: Initilize\nDigitizer: ConfigRealTime\nLJ T7: Initialize\nLJ T7: LoadPinout\nLJ T7: Load355PWMSetting\nLJ T7: Config355PWM\nLJ T7: setDefaultCtrlV\n355 Laser: CheckStatus\n355 Laser: Enable\n355 Laser: CheckStatus\n355 Laser: PWMStart", "State(s) in (\"\")"=w222) -> ("States Out"=w221:string)  [unwired: 13 in]
      }
      frame "Macro: Exit" {
        # "Exit Macro\n(This is called once, when the VI exits)"
        n74 = Unbundle By Name(w224) -> ("Core.Close Panel on Exit?"=w231:bool)
        n75 = Select(t="UI: Front Panel State >> Close", s=w231, f="") -> (s? t:f=w228:string)
        n76 = call <vilib>:"Add State(s) to Queue__JKI_lib_State_Machine.vi"("State(s) in (\"\")"=w228, "State(s) at Back (\"\")"="355 Laser: PWMStop\n355 Laser: Disable\n355 Laser: CheckStatus\nLJ T7: setDefaultCtrlV\nDigitizer: Close\nLJ T7: Close\nData: Cleanup\nExit") -> ("States Out"=w226:string)  [unwired: 13 in]
        n77 = call <vilib>:"Add State(s) to Queue__JKI_lib_State_Machine.vi"("State(s) in Front (\"\")"=w226, "State(s) in (\"\")"=w234) -> ("States Out"=w233:string)  [unwired: 13 in]
        n78 = Bundle By Name(cluster=w224, "Exit Try"=TRUE) -> (w225:T7)
      }
      frame "---------- Digitizer ----------" {
        # "Template Separator\n(You can make a copy of, or modify, this frame)"
        n79 = call <vilib>:"Add State(s) to Queue__JKI_lib_State_Machine.vi"("State(s) in (\"\")"=w238) -> ("States Out"=w237:string)  [unwired: 14 in]
      }
      frame "Digitizer: Select" {
        # "Determin Digitizer\n(You can make a copy of, or modify, this frame)"
        n80 = Unbundle By Name(w239) -> ("Channel"=w244:enum16{"Ch1", "Ch2", "Ch3"})
        n81 = case shown="\"Ch2\"" w244 {
          tunnel: [w251 w255 w259] -> w243
          tunnel: ["0" ("Dig channels") "1" ("Dig channels") "0" ("Dig channels")] -> w241
          tunnel: [w248 w253 w256] -> w240
          tunnel: w239 -> [w249 w252 w257]
          frame "Ch1", Default {
            w251 = refnum<k15> "PXI1Slot3"  # Digitizer
            n82 = Unbundle By Name(w249) -> ("LJ Pins.Ch1 Bias"=w248:string)
          }
          frame "Ch2" {
            w255 = refnum<k15> "PXI1Slot3"  # Digitizer
            n83 = Unbundle By Name(w252) -> ("LJ Pins.Ch2 Bias"=w253:string)
          }
          frame "Ch3" {
            w259 = refnum<k15> "PXI1Slot4"  # Digitizer
            n84 = Unbundle By Name(w257) -> ("LJ Pins.Ch3 Bias"=w256:string)
          }
        }
        n85 = Bundle By Name(cluster=w239, "Digitizer"=w243, "Dig channels"=w241, "LJ pin"=w240) -> (w242:T7)
        n86 = call <vilib>:"Add State(s) to Queue__JKI_lib_State_Machine.vi"("State(s) in (\"\")"=w247) -> ("States Out"=w246:string)  [unwired: 14 in]
      }
      frame "Digitizer: Initilize" {
        # "Initialize Digitizer\n()"
        n87 = Unbundle By Name(w261) -> ("Digitizer"=w260:refnum<k15>)
        n88 = call <instrlib>:"niScope Initialize.vi"("resource name"=w260, "error in"=w262) -> ("error out"=w263:errorcluster)  [unwired: 12 in, 1 out]
        n89 = call <vilib>:"Add State(s) to Queue__JKI_lib_State_Machine.vi"("State(s) in (\"\")"=w265) -> ("States Out"=w264:string)  [unwired: 14 in]
      }
      frame "Digitizer: ConfigMeasurement" {
        w284 = 1200
        w296 = T9 1 items=["AC", "DC", "Ground"] ("vertical coupling")
        # "Template Separator\n(You can make a copy of, or modify, this frame)"
        n90 = Unbundle By Name(w288) -> ("Digitizer"=w276:refnum<k15>, "Dig channels"=w279:string)
        n91 = call <instrlib>:"niScope Acquisition Status.vi"("instrument handle"=w276, "error in"=w275) -> ("instrument handle out"=w286:refnum<k15>, "acquisition status"=w287:i32, "error out"=w285:errorcluster)  [unwired: 11 in]
        n92 = case shown="0, Default" w287 {
          tunnel: w286 -> [w304 w306]
          tunnel: [w301 w306] -> w268
          tunnel: w285 -> [w303 w305]
          tunnel: [w302 w305] -> w273
          frame 0, Default {
            n93 = call <instrlib>:"niScope Abort.vi"("instrument handle"=w304, "error in"=w303) -> ("instrument handle out"=w301:refnum<k15>, "error out"=w302:errorcluster)  [unwired: 12 in]
          }
          frame 1 {
          }
        }
        n94 = property class="niScope"(reference=w268, error in=w273, "Trigger Impedance"=50.0 ("Triggering:Trigger Impedance"), "Active Channel"="0,1", "Vertical Range"=2.0 ("Vertical:Vertical Range"), "Input Impedance"=50.0 ("Vertical:Input Impedance")) -> (reference out=w274:refnum<k15>, error out=w272:errorcluster)
        n95 = call <instrlib>:"niScope Configure Vertical.vi"("instrument handle"=w274, "vertical coupling"=w296, "channels"=w279, "vertical range"=2.0, "vertical offset"=0.5, "error in"=w272, "channel enabled"=TRUE) -> ("instrument handle out"=w295:refnum<k15>, "error out"=w291:errorcluster)  [unwired: 7 in]
        n96 = Bundle By Name(cluster=w288, "num points"=w284) -> (w289:T7)
        n97 = call <instrlib>:"niScope Configure Horizontal Timing.vi"("instrument handle"=w295, "number of records"=5000, "min sample rate"=5000000000.0, "reference position"=0.0, "error in"=w291, "min record length"=w284) -> ("instrument handle out"=w292:refnum<k15>, "error out"=w290:errorcluster)  [unwired: 8 in]
        n98 = call-poly <instrlib>:"niScope Configure Trigger (poly).vi"("instrument handle"=w292, "trigger source"=T3 "VAL_EXTERNAL", "trigger level"=0.5, "error in"=w290) -> ("instrument handle out"=w270:refnum<k15>, "error out"=w269:errorcluster)  [unwired: 10 in]
        n99 = call <instrlib>:"niScope Commit.vi"("instrument handle"=w270, "error in"=w269) -> ("error out"=w281:errorcluster)  [unwired: 12 in, 1 out]
        n100 = call <vilib>:"Add State(s) to Queue__JKI_lib_State_Machine.vi"("State(s) in (\"\")"=w300) -> ("States Out"=w299:string)  [unwired: 14 in]
      }
      frame "Digitizer: ConfigRealTime" {
        w325 = 1200
        w337 = T9 1 items=["AC", "DC", "Ground"] ("vertical coupling")
        # "Template Separator\n(You can make a copy of, or modify, this frame)"
        n101 = Unbundle By Name(w329) -> ("Digitizer"=w317:refnum<k15>, "Dig channels"=w320:string)
        n102 = call <instrlib>:"niScope Acquisition Status.vi"("instrument handle"=w317, "error in"=w316) -> ("instrument handle out"=w327:refnum<k15>, "acquisition status"=w328:i32, "error out"=w326:errorcluster)  [unwired: 11 in]
        n103 = case shown="0, Default" w328 {
          tunnel: w327 -> [w345 w347]
          tunnel: [w342 w347] -> w309
          tunnel: w326 -> [w344 w346]
          tunnel: [w343 w346] -> w314
          frame 0, Default {
            n104 = call <instrlib>:"niScope Abort.vi"("instrument handle"=w345, "error in"=w344) -> ("instrument handle out"=w342:refnum<k15>, "error out"=w343:errorcluster)  [unwired: 12 in]
          }
          frame 1 {
          }
        }
        n105 = property class="niScope"(reference=w309, error in=w314, "Trigger Impedance"=50.0 ("Triggering:Trigger Impedance"), "Active Channel"="0,1", "Vertical Range"=2.0 ("Vertical:Vertical Range"), "Input Impedance"=50.0 ("Vertical:Input Impedance")) -> (reference out=w315:refnum<k15>, error out=w313:errorcluster)
        n106 = call <instrlib>:"niScope Configure Vertical.vi"("instrument handle"=w315, "vertical coupling"=w337, "channels"=w320, "vertical range"=2.0, "vertical offset"=0.5, "error in"=w313, "channel enabled"=TRUE) -> ("instrument handle out"=w336:refnum<k15>, "error out"=w332:errorcluster)  [unwired: 7 in]
        n107 = Bundle By Name(cluster=w329, "num points"=w325) -> (w330:T7)
        n108 = call <instrlib>:"niScope Configure Horizontal Timing.vi"("instrument handle"=w336, "number of records"=1, "min sample rate"=5000000000.0, "reference position"=0.0, "error in"=w332, "min record length"=w325) -> ("instrument handle out"=w333:refnum<k15>, "error out"=w331:errorcluster)  [unwired: 8 in]
        n109 = call-poly <instrlib>:"niScope Configure Trigger (poly).vi"("instrument handle"=w333, "trigger source"=T3 "VAL_EXTERNAL", "trigger level"=0.5, "error in"=w331) -> ("instrument handle out"=w311:refnum<k15>, "error out"=w310:errorcluster)  [unwired: 10 in]
        n110 = call <instrlib>:"niScope Commit.vi"("instrument handle"=w311, "error in"=w310) -> ("error out"=w322:errorcluster)  [unwired: 12 in, 1 out]
        n111 = call <vilib>:"Add State(s) to Queue__JKI_lib_State_Machine.vi"("State(s) in (\"\")"=w341) -> ("States Out"=w340:string)  [unwired: 14 in]
      }
      frame "Digitizer: Acquire" {
        # "Template Separator\n(You can make a copy of, or modify, this frame)"
        n112 = Unbundle By Name(w356) -> ("Digitizer"=w352:refnum<k15>, "Dig channels"=w355:string, "num points"=w354:i32)
        n113 = call <instrlib>:"niScope Acquisition Status.vi"("instrument handle"=w352, "error in"=w350) -> ("instrument handle out"=w349:refnum<k15>, "acquisition status"=w348:i32, "error out"=w351:errorcluster)  [unwired: 11 in]
        n114 = case shown="1" w348 {
          tunnel: w355 -> [_ w366]
          tunnel: w354 -> [_ w364]
          tunnel: [w359 w363] -> w353
          tunnel: w351 -> [w359 w361]
          tunnel: w349 -> [_ w360]
          frame 0, Default {
          }
          frame 1 {
            n115 = call <instrlib>:"niScope Initiate Acquisition.vi"("instrument handle"=w360, "error in"=w361) -> ("instrument handle out"=w367:refnum<k15>, "error out"=w365:errorcluster)  [unwired: 12 in]
            n116 = call-poly <instrlib>:"niScope Fetch (poly).vi"("error in"=w365, "numSamples"=w364, "channels"=w366, "instrument handle"=w367) -> ("error out"=w363:errorcluster, "wfm"=→"Waveform Graph":dbl[])  [unwired: 4 in, 2 out]
          }
        }
        n117 = call <vilib>:"Add State(s) to Queue__JKI_lib_State_Machine.vi"("State(s) in (\"\")"=w358) -> ("States Out"=w357:string)  [unwired: 14 in]
      }
      frame "Digitizer: Close" {
        # "Template Separator\n(You can make a copy of, or modify, this frame)"
        n118 = Unbundle By Name(w373) -> ("Digitizer"=w372:refnum<k15>)
        n119 = call <instrlib>:"niScope Abort.vi"("instrument handle"=w372, "error in"=w368) -> ("instrument handle out"=w371:refnum<k15>, "error out"=w370:errorcluster)  [unwired: 12 in]
        n120 = call <instrlib>:"niScope Close.vi"("instrument handle"=w371, "error in"=w370) -> ("error out"=w369:errorcluster)  [unwired: 13 in]
        n121 = call <vilib>:"Add State(s) to Queue__JKI_lib_State_Machine.vi"("State(s) in (\"\")"=w375) -> ("States Out"=w374:string)  [unwired: 14 in]
      }
      frame "---------- LJ T7 ----------" {
        # "Template Separator\n(You can make a copy of, or modify, this frame)"
        n122 = call <vilib>:"Add State(s) to Queue__JKI_lib_State_Machine.vi"("State(s) in (\"\")"=w379) -> ("States Out"=w378:string)  [unwired: 14 in]
      }
      frame "LJ T7: Load355PWMSetting" {
        # "Template Separator\n(You can make a copy of, or modify, this frame)"
        n123 = call <userlib>:"Current VIs Parent Directory__ogtk.vi"() -> ("Parent Directory (+ Relative)"=w385:path)  [unwired: 5 in]
        n124 = Build Path(base path=w385, name or relative path="SubVI\\LabJack\\PWM_setting_355.config") -> (appended path=w383:path)
        n125 = call "ReadPWMConfig(SubVI).vi"("appended path"=w383) -> ("PWM Setting"=w380:T6)  [unwired: 9 in, 1 out]
        n126 = call <vilib>:"Add State(s) to Queue__JKI_lib_State_Machine.vi"("State(s) in (\"\")"=w388) -> ("States Out"=w387:string)  [unwired: 14 in]
        n127 = Bundle By Name(cluster=w381, "PWM Setting"=w380) -> (w382:T7)
      }
      frame "LJ T7: Config355PWM" {
        w393 = 0.0 ("element")
        w409 = "DIO_EF_CLOCK1_ENABLE"
        # "Template Separator\n(You can make a copy of, or modify, this frame)"
        n128 = Unbundle By Name(w389) -> ("PWM Setting.DIO_EF_CLOCK1_DIVISOR"=w402:i16, "PWM Setting.DIO_EF_CLOCK1_ROLL_VALUE"=w401:i32, "PWM Setting.DIO#_EF_INDEX"=w398:i16, "PWM Setting.DIO#_EF_OPTIONS"=w397:i16, "PWM Setting.DIO#_EF_CONFIG_A"=w396:i32)
        n129 = Unbundle By Name(w389) -> ("LJ Pins.355 PWM"=w408:string)
        n130 = Unbundle By Name(w389) -> ("LJ Handle"=w390:i32)
        n131 = Concatenate Strings(w408, "_EF_ENABLE" ("string")) -> (w404:string)
        n132 = Concatenate Strings(w408, "_EF_INDEX") -> (w407:string)
        n133 = Concatenate Strings(w408, "_EF_OPTIONS") -> (w406:string)
        n134 = Concatenate Strings(w408, "_EF_CONFIG_A") -> (w405:string)
        n135 = Build Array(w393, w393, w402, w401, 1.0 ("element"), 0.0 ("element"), w398, w397, w396) -> (w395:dbl[])
        n136 = call <vilib>:"Add State(s) to Queue__JKI_lib_State_Machine.vi"("State(s) in (\"\")"=w417) -> ("States Out"=w416:string)  [unwired: 14 in]
        n137 = Build Array("DIO_EF_CLOCK0_ENABLE", w409, "DIO_EF_CLOCK1_DIVISOR", "DIO_EF_CLOCK1_ROLL_VALUE", w409, w404, w407, w406, w405) -> (w403:string[])
        n138 = call <vilib>:"LJM_eWriteNames.vi"("Handle In"=w390, "aNames"=w403, "aValuesIn"=w395, "error in"=w392) -> ("error out"=w391:errorcluster)  [unwired: 9 in, 2 out]
      }
      frame "LJ T7: Initialize" {
        # "Template Separator\n(You can make a copy of, or modify, this frame)"
        n139 = call "LJ_Open.vi"("error in"=w421) -> ("error out"=w422:errorcluster, "Handle Out"=w418:i32)  [unwired: 8 in, 1 out]
        n140 = Bundle By Name(cluster=w419, "LJ Handle"=w418) -> (w420:T7)
        n141 = call <vilib>:"Add State(s) to Queue__JKI_lib_State_Machine.vi"("State(s) in (\"\")"=w424) -> ("States Out"=w423:string)  [unwired: 14 in]
      }
      frame "LJ T7: LoadPinout" {
        # "Template Separator\n(You can make a copy of, or modify, this frame)"
        n142 = call <userlib>:"Current VIs Parent Directory__ogtk.vi"() -> ("Parent Directory (+ Relative)"=w430:path)  [unwired: 5 in]
        n143 = Build Path(base path=w430, name or relative path="SubVI\\LabJack\\LJ_pin_setting.config") -> (appended path=w428:path)
        n144 = call "ReadLabjackConfig(SubVI).vi"("appended path"=w428) -> ("Utility"=w425:T5)  [unwired: 9 in, 1 out]
        n145 = call <vilib>:"Add State(s) to Queue__JKI_lib_State_Machine.vi"("State(s) in (\"\")"=w433) -> ("States Out"=w432:string)  [unwired: 14 in]
        n146 = Bundle By Name(cluster=w426, "LJ Pins"=w425) -> (w427:T7)
      }
      frame "LJ T7: setDefaultCtrlV" {
        # "Template Separator\n(You can make a copy of, or modify, this frame)"
        n147 = Unbundle By Name(w439) -> ("LJ Handle"=w438:i32, "LJ pin"=w437:string)
        n148 = call <vilib>:"LJM_eWriteName.vi"("Handle In"=w438, "Name"=w437, "Value"=0.0, "error in"=w434) -> ("error out"=w435:errorcluster)  [unwired: 10 in, 1 out]
        n149 = call <vilib>:"Add State(s) to Queue__JKI_lib_State_Machine.vi"("State(s) in (\"\")"=w441) -> ("States Out"=w440:string)  [unwired: 14 in]
      }
      frame "LJ T7: Close" {
        # "Template Separator\n(You can make a copy of, or modify, this frame)"
        n150 = Unbundle By Name(w445) -> ("LJ Handle"=w444:i32)
        n151 = call <vilib>:"LJM_Close.vi"("error in"=w442, "Handle"=w444) -> ("error out"=w443:errorcluster)  [unwired: 9 in]
        n152 = call <vilib>:"Add State(s) to Queue__JKI_lib_State_Machine.vi"("State(s) in (\"\")"=w447) -> ("States Out"=w446:string)  [unwired: 14 in]
      }
      frame "---------- iRFData ----------" {
        # "Template Separator\n(You can make a copy of, or modify, this frame)"
        n153 = call <vilib>:"Add State(s) to Queue__JKI_lib_State_Machine.vi"("State(s) in (\"\")"=w451) -> ("States Out"=w450:string)  [unwired: 14 in]
      }
      frame "iRFData: Acquire" {
        # "Template Separator\n(You can make a copy of, or modify, this frame)"
        n154 = Unbundle By Name(w461) -> ("Digitizer"=w467:refnum<k15>, "Dig channels"=w466:string, "num points"=w465:i32)  [unwired: 2 out]
        n155 = call <userlib>:"Wait (ms)__ogtk.vi"("error in (no error)"=w464, "milliseconds to wait"=u32 100) -> ("error out"=w458:errorcluster)  [unwired: 8 in, 1 out]
        n156 = local read "Current V"() -> (w455:dbl)
        n157 = call <instrlib>:"niScope Initiate Acquisition.vi"("instrument handle"=w467, "error in"=w458) -> ("instrument handle out"=w460:refnum<k15>, "error out"=w459:errorcluster)  [unwired: 12 in]
        n158 = call <vilib>:"Add State(s) to Queue__JKI_lib_State_Machine.vi"("State(s) in Front (\"\")"="Digitizer: ConfigRealTime" ("State(s) in Front (\"\")"), "State(s) in (\"\")"=w469) -> ("States Out"=w468:string)  [unwired: 13 in]
        n159 = call-poly <instrlib>:"niScope Fetch (poly).vi"("timeout"=10.5, "error in"=w459, "numSamples"=w465, "channels"=w466, "instrument handle"=w460) -> ("error out"=w463:errorcluster, "wfm"=w454:dbl[][])  [unwired: 3 in, 2 out]
        n160 = Bundle By Name(cluster=w461, "V"=w455, "wfm"=w454) -> (w462:T7)
        n161 = Index Array(array=w454) -> (element=w453:dbl[])  [unwired: 2 in]
        n162 = local write "Waveform Graph"(w453) -> ()
      }
      frame "iRFData: Save" {
        # "Template Separator\n(You can make a copy of, or modify, this frame)"
        n163 = Unbundle By Name(w479) -> ("Channel"=w478:enum16{"Ch1", "Ch2", "Ch3"})
        n164 = case shown="\"Ch3\"" w478 {
          tunnel: ["Ch1" "Ch2" "Ch3"] -> w477
          frame "Ch1", Default {
          }
          frame "Ch2" {
          }
          frame "Ch3" {
          }
        }
        n165 = local read "Current V"() -> (w474:dbl)
        n166 = Current VI's Path() -> (path=w482:path)
        n167 = Number To Fractional String(number=w474, precision (6)=i16 2) -> (F-format string=w473:string)  [unwired: 2 in]
        n168 = Concatenate Strings("Prefix", w477, "_iRF" ("default name"), w473, "Suffix") -> (w475:string)
        n169 = call "File Dialog"("start path"=w482, "default name"=w475) -> ("selected path"=w483:path)  [unwired: 10 in, 3 out]
        n170 = Unbundle By Name(w479) -> ("V"=w481:dbl, "wfm"=w493:dbl[][])
        n171 = TDMS Open(8:w484, 10:T4."create or replace" ("operation (0:open)"), 11:w483) -> (0:w496:errorcluster, 3:w499:refnum<k34>)  [unwired: 4 in]
        n172 = Array Size(array=w493) -> (size(s)=w497:i32[])
        n173 = TDMS Set Properties(5:w497, 7:string[] ["Num of points", "Data Length"] ("property names"), 8:w496, 11:w499) -> (0:w494:errorcluster, 3:w495:refnum<k34>)  [unwired: 2 in, 2 out]
        n174 = for {
          tunnel: w493 -> [w507] mode=indexing
          tunnel: [w507] -> w492 mode=concatenating
          tunnel: w481 -> [w506]
          tunnel: [w506] -> w480 mode=indexing
          # "Reshape"
        }
        n175 = TDMS Write(0:w495, 7:string[] ["Waveform"] ("channel name(s) in (Untitled)"), 9:w492, 11:w494) -> (4:w490:refnum<k34>, 15:w489:errorcluster)  [unwired: 2 in, 2 out]
        n176 = TDMS Write(0:w490, 7:string[] ["CtrlV"] ("channel name(s) in (Untitled)"), 9:w480, 11:w489) -> (4:w487:refnum<k34>, 15:w486:errorcluster)  [unwired: 2 in, 2 out]
        n177 = call <vilib>:"Add State(s) to Queue__JKI_lib_State_Machine.vi"("State(s) in (\"\")"=w502) -> ("States Out"=w501:string)  [unwired: 14 in]
        n178 = TDMS Close(8:w486, 11:w487) -> (0:w485:errorcluster)  [unwired: 1 out]
      }
      frame "---------- 355 Laser ----------" {
        # "Template Separator\n(You can make a copy of, or modify, this frame)"
        n179 = call <vilib>:"Add State(s) to Queue__JKI_lib_State_Machine.vi"("State(s) in (\"\")"=w511) -> ("States Out"=w510:string)  [unwired: 14 in]
      }
      frame "355 Laser: CheckStatus" {
        # "if average < 1, laser on\nif average > 9, laser off\nif 1<average<9, interlock open, blink indicator"
        # "take 10 measuremt and look at average"
        # "Template Separator\n(You can make a copy of, or modify, this frame)"
        n180 = Unbundle By Name(w514) -> ("LJ Handle"=w512:i32, "LJ Pins.Laser Ready"=w521:string)
        n181 = for {
          N: 10 -> [_]
          tunnel: w512 -> [w551]
          tunnel: w521 -> [w550]
          shift-right: [w549] -> w519
          shift-left: w516 -> [w548]
          tunnel: [w546] -> w517 mode=indexing
          n182 = call <vilib>:"LJM_eReadName.vi"("Handle In"=w551, "Name"=w550, "error in"=w548) -> ("Value"=w546:dbl, "error out"=w549:errorcluster)  [unwired: 10 in, 1 out]
          n183 = Wait (ms)(milliseconds to wait=u32 50) -> ()  [unwired: 1 out]
        }
        n184 = case shown="No Error" w519 {
          selector: w519 -> [w528 w544]
          tunnel: [w530 FALSE] -> w513
          tunnel: [w529 w544] -> _
          tunnel: [w524 nan] -> w518
          tunnel: w517 -> [w526 _]
          frame No Error {
            n185 = call-poly <vilib>:"Mean.vi"("X"=w526) -> ("mean"=w524:dbl)  [unwired: 1 out]
            n186 = Less?(x=w524, y=2.0) -> (x < y?=w525:bool)
            n187 = case shown="False" w525 {
              tunnel: [w533 TRUE] -> w530
              tunnel: w524 -> [w536 _]
              tunnel: w528 -> [w532 w541]
              tunnel: [w531 w541] -> w529
              frame False {
                n188 = Greater?(x=w536, y=9.0) -> (0:w534:bool)
                n189 = case shown="True" w534 {
                  tunnel: [FALSE FALSE] -> w533
                  tunnel: w532 -> [_ w539]
                  tunnel: [errorcluster {"status"=TRUE, "code"=5002, "source"="355 Laser"} ("error out") w539] -> w531
                  frame False {
                  }
                  frame True {
                  }
                }
              }
              frame True {
              }
            }
          }
          frame Error {
          }
        }
        "laser EM lamp V" <- w518
        "355nm Laser" <- w513
        n190 = call <vilib>:"Add State(s) to Queue__JKI_lib_State_Machine.vi"("State(s) in (\"\")"=w523) -> ("States Out"=w522:string)  [unwired: 14 in]
        n191 = Bundle By Name(cluster=w514, "355 Status"=w513) -> (w515:T7)
      }
      frame "355 Laser: PWMStart" {
        # "Template Separator\n(You can make a copy of, or modify, this frame)"
        n192 = Unbundle By Name(w555) -> ("LJ Pins.355 PWM"=w559:string, "LJ Handle"=w554:i32)
        n193 = Concatenate Strings(w559, "_EF_ENABLE" ("string")) -> (w557:string)
        n194 = call <vilib>:"LJM_eWriteName.vi"("Handle In"=w554, "Name"=w557, "Value"=1.0, "error in"=w552) -> ("error out"=w553:errorcluster)  [unwired: 10 in, 1 out]
        n195 = call <vilib>:"Add State(s) to Queue__JKI_lib_State_Machine.vi"("State(s) in (\"\")"=w561) -> ("States Out"=w560:string)  [unwired: 14 in]
      }
      frame "355 Laser: PWMStop" {
        # "Template Separator\n(You can make a copy of, or modify, this frame)"
        n196 = Unbundle By Name(w565) -> ("LJ Pins.355 PWM"=w569:string, "LJ Handle"=w564:i32)
        n197 = Concatenate Strings(w569, "_EF_ENABLE" ("string")) -> (w567:string)
        n198 = call <vilib>:"LJM_eWriteName.vi"("Handle In"=w564, "Name"=w567, "Value"=0.0, "error in"=w562) -> ("error out"=w563:errorcluster)  [unwired: 10 in, 1 out]
        n199 = call <vilib>:"Add State(s) to Queue__JKI_lib_State_Machine.vi"("State(s) in (\"\")"=w571) -> ("States Out"=w570:string)  [unwired: 14 in]
      }
      frame "355 Laser: Enable" {
        # "Template Separator\n(You can make a copy of, or modify, this frame)"
        n200 = Unbundle By Name(w576) -> ("LJ Pins.Laser Start/Stop"=w578:string, "355 Status"=w577:bool, "LJ Handle"=w575:i32)
        n201 = case shown="False" w577 {
          tunnel: w578 -> [w588 _]
          tunnel: [w583 w592] -> w573
          tunnel: w575 -> [w582 _]
          tunnel: w574 -> [w581 w592]
          frame False {
            n202 = call <vilib>:"LJM_eWriteName.vi"("Handle In"=w582, "Name"=w588, "Value"=1.0, "error in"=w581) -> ("Handle Out"=w589:i32, "error out"=w587:errorcluster)  [unwired: 10 in]
            n203 = call <userlib>:"Wait (ms)__ogtk.vi"("error in (no error)"=w587, "milliseconds to wait"=u32 250) -> ("error out"=w586:errorcluster)  [unwired: 8 in, 1 out]
            n204 = call <vilib>:"LJM_eWriteName.vi"("Handle In"=w589, "Name"=w588, "Value"=0.0, "error in"=w586) -> ("error out"=w584:errorcluster)  [unwired: 10 in, 1 out]
            n205 = call <userlib>:"Tick Count (ms)__ogtk.vi"("error in (no error)"=w584) -> ("error out"=w583:errorcluster)  [unwired: 9 in, 1 out]
          }
          frame True {
            (unwired) u32 0 ("millisecond timer value")
          }
        }
        n206 = call <vilib>:"Add State(s) to Queue__JKI_lib_State_Machine.vi"("State(s) in (\"\")"=w580) -> ("States Out"=w579:string)  [unwired: 14 in]
        n207 = Wait (ms)(milliseconds to wait=u32 5000) -> ()  [unwired: 1 out]
      }
      frame "355 Laser: Disable" {
        # "Template Separator\n(You can make a copy of, or modify, this frame)"
        n208 = Unbundle By Name(w596) -> ("LJ Pins.Laser Start/Stop"=w598:string, "355 Status"=w597:bool, "LJ Handle"=w595:i32)
        n209 = case shown="False" w597 {
          tunnel: w598 -> [_ w609]
          tunnel: [w601 w603] -> w594
          tunnel: w595 -> [_ w604]
          tunnel: w593 -> [w601 w602]
          frame False {
            (unwired) u32 0 ("millisecond timer value")
          }
          frame True {
            n210 = call <vilib>:"LJM_eWriteName.vi"("Handle In"=w604, "Name"=w609, "Value"=1.0, "error in"=w602) -> ("Handle Out"=w610:i32, "error out"=w608:errorcluster)  [unwired: 10 in]
            n211 = call <userlib>:"Wait (ms)__ogtk.vi"("error in (no error)"=w608, "milliseconds to wait"=u32 250) -> ("error out"=w607:errorcluster)  [unwired: 8 in, 1 out]
            n212 = call <vilib>:"LJM_eWriteName.vi"("Handle In"=w610, "Name"=w609, "Value"=0.0, "error in"=w607) -> ("error out"=w605:errorcluster)  [unwired: 10 in, 1 out]
            n213 = call <userlib>:"Tick Count (ms)__ogtk.vi"("error in (no error)"=w605) -> ("error out"=w603:errorcluster)  [unwired: 9 in, 1 out]
          }
        }
        n214 = call <vilib>:"Add State(s) to Queue__JKI_lib_State_Machine.vi"("State(s) in (\"\")"=w600) -> ("States Out"=w599:string)  [unwired: 14 in]
      }
      frame "---------- New Category ----------" {
        # "Template Separator\n(You can make a copy of, or modify, this frame)"
        n215 = call <vilib>:"Add State(s) to Queue__JKI_lib_State_Machine.vi"("State(s) in (\"\")"=w616) -> ("States Out"=w615:string)  [unwired: 14 in]
      }
      frame "New Category: 1" {
        # "Your code here.\n(You can make a copy of, or modify, this frame)"
        n216 = call <vilib>:"Add State(s) to Queue__JKI_lib_State_Machine.vi"("State(s) in (\"\")"=w620) -> ("States Out"=w619:string)  [unwired: 14 in]
      }
      frame "New Category: 2" {
        # "Your code here.\n(You can make a copy of, or modify, this frame)"
        n217 = call <vilib>:"Add State(s) to Queue__JKI_lib_State_Machine.vi"("State(s) in (\"\")"=w624) -> ("States Out"=w623:string)  [unwired: 14 in]
      }
    }
  }
  "error out" <- w1
